vi "Dac_Output_cam_trig_multiple_digital_signals.vi"(0 "File to read":path=path "C:/Users/lpk27/Documents/pan-ASLMsynched/pan-ASLM/Calibration files/newcalibration_voice coil input_25msflyback.txt", 1 "Image acquisition time (ms)":dbl=1000.0, 2 "Delay between frames":dbl=25.0, 3 "Laser Toggles":T1 {"Laser 488 order selection" items=["Not active", "1", "2", "3", "4"]; "Laser 642 order selection" items=["Not active", "1", "2", "3", "4"]; "Laser 595 order selection" items=["Not active", "1", "2", "3", "4"]; "Laser 560 order selection" items=["Not active", "1", "2", "3", "4"]; "Laser 642 nm power" min=0.0 max=5.0 scale=0.0..100.0; "Laser 595 nm power" min=0.0 max=5.0 scale=0.0..100.0; "Laser 560 nm power" min=0.0 max=5.0 scale=0.0..100.0; "Laser 488 nm power" min=0.0 max=5.0 scale=0.0..100.0}, 4 "stop":bool, 5 "error in":errorcluster, 6 "Time Target (s)":dbl=-1.0, 11 "Setup":enum16{"Test setup", "Microscope"}(ring)) -> (19 "error out":errorcluster)   [LabVIEW 2020]
uses:
  typedefs/Laser_toggles_typedef.ctl
  <vilib>/DAQmx/write.llb/DAQmx Write (Digital Wfm 1Chan NSamp).vi
  <vilib>/DAQmx/write.llb/DAQmx Write (Analog Wfm 1Chan NSamp).vi
  <vilib>/Utility/file.llb/Read Delimited Spreadsheet (DBL).vi
  <vilib>/DAQmx/create/channels.llb/DAQmx Create Channel (AO-Voltage-Basic).vi
  <vilib>/DAQmx/configure/timing.llb/DAQmx Timing (Sample Clock).vi
  <vilib>/DAQmx/miscellaneous.llb/DAQmx Fill In Error Info.vi
  <vilib>/DAQmx/create/channels.llb/DAQmx Create Channel (CO-Pulse Generation-Ticks).vi
  <vilib>/DAQmx/configure/timing.llb/DAQmx Timing (Implicit).vi
  <vilib>/DAQmx/create/channels.llb/DAQmx Create Channel (DO-Digital Output).vi
  <vilib>/Waveform/DWDTOps.llb/DWDT Uncompress Digital.vi
  <vilib>/DAQmx/create/channels.llb/DAQmx Create Channel (CO-Pulse Generation-Frequency).vi
  Global stop DAQ.vi
  <resource>/objmgr/daqmx.rc
panel:
  out "error out 4":errorcluster
  out "error out 3":errorcluster
  out "error out 2":errorcluster
  out "Digital Waveform Graph":digitalwaveform(graph)
  out "LabVIEW generated Sawtooth input (blue) and Camera trigger (red)":waveform(dbl)(graph)={"t0"=timestamp(0 s since 1904-01-01), "dt"=1.0, "Y"=array[3075 elements]}
  out "# Samples written per channel":u32=3075
  out "actual frequency":dbl=1000.0
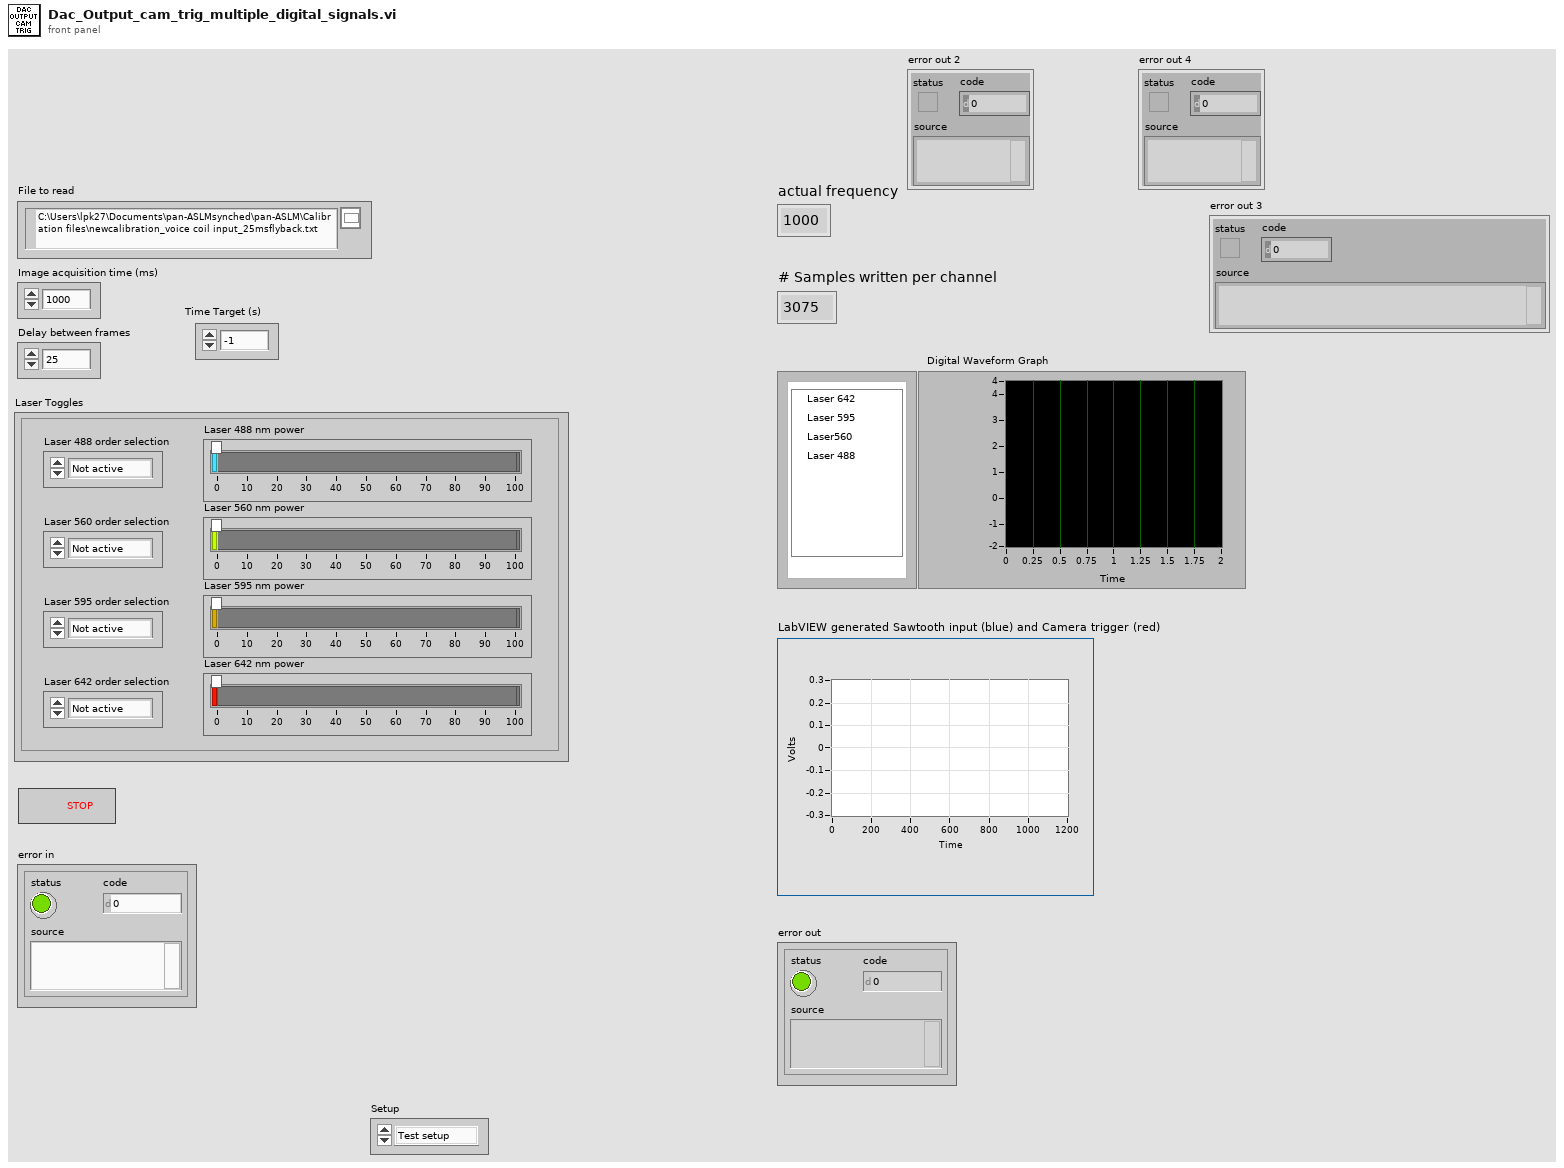
[diagram p1: front panel]
types:
  T1 = typedef "Laser_toggles_typedef.ctl" = cluster{"Laser 488 nm power":dbl, "Laser 560 nm power":dbl, "Laser 595 nm power":dbl, "Laser 642 nm power":dbl, "Laser 560 order selection":u16, "Laser 595 order selection":u16, "Laser 642 order selection":u16, "Laser 488 order selection":u16}
  T2 = typedef "DAQ_channel_typedef.ctl" = cluster{"CO.Pulse.Term":tag, "Voice coil analog output":tag, "counter":tag, "CO.Pulse.Term 2":tag, "AOTF lines":tag, "counter 2":tag, "CO.Pulse.Term 3":tag, "counter 3":tag}
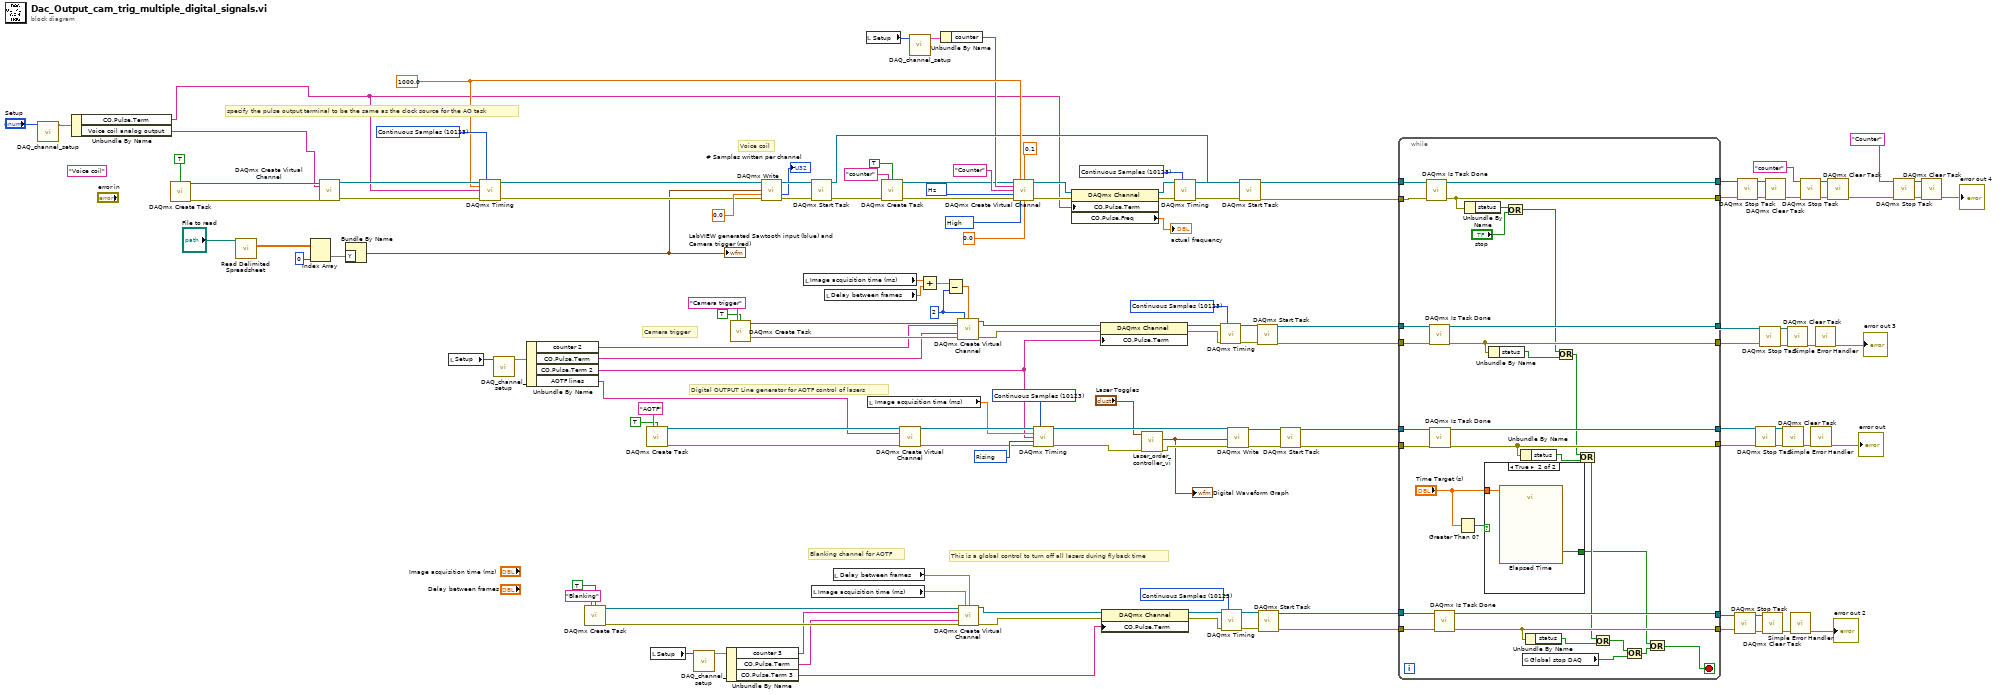
[diagram p0: block diagram]
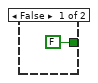
[diagram p2: hidden frame]
diagram:
  (unwired) "Voice coil" ("new task name")
  w86 = 10123 items=["Finite Samples"=10178, "Continuous Samples"=10123, "Hardware Timed Single Point"=12522] ("sample mode")
  w91 = 10123 items=["Finite Samples"=10178, "Continuous Samples"=10123, "Hardware Timed Single Point"=12522] ("sample mode")
  w99 = 10280 items=["Rising"=10280, "Falling"=10171] ("active edge")
  w71 = u32 2 ("high ticks")
  w109 = 10123 items=["Finite Samples"=10178, "Continuous Samples"=10123, "Hardware Timed Single Point"=12522] ("sample mode")
  w121 = 10192 items=["High"=10192, "Low"=10214] ("idle state")
  w122 = 10373 items=["Hz"=10373] ("units")
  w115 = 10123 items=["Finite Samples"=10178, "Continuous Samples"=10123, "Hardware Timed Single Point"=12522] ("sample mode")
  w114 = 1000.0 ("rate")
  w136 = 10123 items=["Finite Samples"=10178, "Continuous Samples"=10123, "Hardware Timed Single Point"=12522] ("sample mode")
  # "This is a global control to turn off all lasers during flyback time"
  # "Voice coil"
  # "Camera trigger"
  # "Digital OUTPUT Line generator for AOTF control of lasers"
  # "Blanking channel for AOTF"
  # "specify the pulse output terminal to be the same as the clock source for the AO task"
  n1 = call "DAQ_channel_setup.vi"("Text Ring"="Setup") -> ("DAQ channels OUT"=w24:T2)  [unwired: 10 in]
  n2 = Unbundle By Name(w24) -> ("CO.Pulse.Term"=w9:tag, "Voice coil analog output"=w25:tag)
  n3 = call <vilib>:"DAQmx Create Task.vi"("auto cleanup"=TRUE) -> ("task out"=w63:refnum<k21>, "error out"=w62:errorcluster)  [unwired: 13 in]
  n4 = call-poly <vilib>:"Read Delimited Spreadsheet.vi"("file path (dialog if empty)"="File to read") -> ("all rows"=w105:dbl[][])  [unwired: 9 in, 5 out]
  n5 = Index Array(array=w105, index (col)=0 ("disabled index (col)")) -> (element=w103:dbl[])  [unwired: 1 in]
  n6 = call-poly <vilib>:"DAQmx Create Virtual Channel.vi"("task in"=w63, "physical channels"=w25, "error in"=w62) -> ("task out"=w138:refnum<k21>, "error out"=w137:errorcluster)  [unwired: 11 in]
  n7 = Bundle By Name("Y"=w103) -> (w102:waveform(dbl))  [unwired: 1 in]
  "LabVIEW generated Sawtooth input (blue) and Camera trigger (red)" <- w102
  n8 = local read "Setup"() -> (w12:enum16{"Test setup", "Microscope"})
  n9 = call-poly <vilib>:"DAQmx Timing.vi"("task/channels in"=w138, "sample mode"=w136, "rate"=w114, "source"=w9, "error in"=w137) -> ("task out"=w117:refnum<k21>, "error out"=w116:errorcluster)  [unwired: 9 in]
  n10 = call "DAQ_channel_setup.vi"("Text Ring"=w12) -> ("DAQ channels OUT"=w21:T2)  [unwired: 10 in]
  n11 = Unbundle By Name(w21) -> ("counter 2"=w15:tag, "CO.Pulse.Term"=w5:tag, "CO.Pulse.Term 2"=w20:tag, "AOTF lines"=w19:tag)
  n12 = call <vilib>:"DAQmx Create Task.vi"("new task name"="Blanking", "auto cleanup"=TRUE) -> ("task out"=w68:refnum<k21>, "error out"=w67:errorcluster)  [unwired: 12 in]
  n13 = call <vilib>:"DAQmx Create Task.vi"("new task name"="AOTF", "auto cleanup"=TRUE) -> ("task out"=w65:refnum<k21>, "error out"=w64:errorcluster)  [unwired: 12 in]
  n14 = local read "Setup"() -> (w13:enum16{"Test setup", "Microscope"})
  n15 = call "DAQ_channel_setup.vi"("Text Ring"=w13) -> ("DAQ channels OUT"=w18:T2)  [unwired: 10 in]
  n16 = Unbundle By Name(w18) -> ("counter 3"=w17:tag, "CO.Pulse.Term"=w4:tag, "CO.Pulse.Term 3"=w16:tag)
  n17 = call <vilib>:"DAQmx Create Task.vi"("new task name"="Camera trigger", "auto cleanup"=TRUE) -> ("task out"=w59:refnum<k21>, "error out"=w60:errorcluster)  [unwired: 12 in]
  n18 = call-poly <vilib>:"DAQmx Write.vi"("task/channels in"=w117, "data"=w102, "timeout"=0.0, "error in"=w116) -> ("task out"=w126:refnum<k21>, "number of samples written per channel"=→"# Samples written per channel":u32, "error out"=w125:errorcluster)  [unwired: 9 in]
  n19 = local read "Image acquisition time (ms)"() -> (w74:dbl)
  n20 = call <vilib>:"DAQmx Start Task.vi"("task/channels in"=w126, "error in"=w125) -> ("task out"=w30:refnum<k21>, "error out"=w120:errorcluster)  [unwired: 12 in]
  n21 = local read "Image acquisition time (ms)"() -> (w76:dbl)
  n22 = local read "Delay between frames"() -> (w73:dbl)
  n23 = local read "Delay between frames"() -> (w75:dbl)
  n24 = local read "Setup"() -> (w11:enum16{"Test setup", "Microscope"})
  n25 = local read "Image acquisition time (ms)"() -> (w81:dbl)
  n26 = call <vilib>:"DAQmx Create Task.vi"("new task name"="counter", "auto cleanup"=TRUE, "error in"=w120) -> ("task out"=w7:refnum<k21>, "error out"=w133:errorcluster)  [unwired: 11 in]
  n27 = call-poly <vilib>:"DAQmx Create Virtual Channel.vi"("task in"=w65, "lines"=w19, "error in"=w64) -> ("task out"=w98:refnum<k21>, "error out"=w97:errorcluster)  [unwired: 11 in]
  n28 = call "DAQ_channel_setup.vi"("Text Ring"=w11) -> ("DAQ channels OUT"=w23:T2)  [unwired: 10 in]
  n29 = Add(x=w74, y=w73) -> (x+y=w72:dbl)
  n30 = Unbundle By Name(w23) -> ("counter"=w22:tag)
  n31 = Subtract(x=w72, y=w71) -> (x-y=w70:dbl)
  n32 = call-poly <vilib>:"DAQmx Create Virtual Channel.vi"("task in"=w59, "high ticks"=w71, "low ticks"=w70, "counter"=w15, "source of ticks"=w5, "error in"=w60) -> ("task out"=w113:refnum<k21>, "error out"=w101:errorcluster)  [unwired: 8 in]
  n33 = call-poly <vilib>:"DAQmx Create Virtual Channel.vi"("task in"=w68, "high ticks"=w76, "low ticks"=w75, "counter"=w17, "source of ticks"=w4, "error in"=w67) -> ("task out"=w90:refnum<k21>, "error out"=w83:errorcluster)  [unwired: 8 in]
  n34 = call-poly <vilib>:"DAQmx Create Virtual Channel.vi"("task in"=w7, "frequency"=w114, "duty cycle"=0.1, "counter"=w22, "name to assign"="Counter", "units"=w122, "error in"=w133, "idle state"=w121, "initial delay"=0.0) -> ("task out"=w132:refnum<k21>, "error out"=w131:errorcluster)  [unwired: 5 in]
  n35 = call-poly <vilib>:"DAQmx Timing.vi"("task/channels in"=w98, "sample mode"=w91, "rate"=w81, "source"=w20, "active edge"=w99, "error in"=w97) -> ("task out"=w94:refnum<k21>, "error out"=w79:errorcluster)  [unwired: 8 in]
  n36 = property class="DAQmx Channel"(reference=w132, error in=w131, "CO.Pulse.Term"=w9) -> (reference out=w128:refnum<k21>, error out=w129:errorcluster, "CO.Pulse.Freq"=→"actual frequency":dbl)
  n37 = property class="DAQmx Channel"(reference=w113, error in=w101, "CO.Pulse.Term"=w20) -> (reference out=w100:refnum<k21>, error out=w110:errorcluster)
  n38 = property class="DAQmx Channel"(reference=w90, error in=w83, "CO.Pulse.Term"=w16) -> (reference out=w82:refnum<k21>, error out=w87:errorcluster)
  n39 = call "Laser_order_controller_vi.vi"("error in"=w79, "Laser Toggles"="Laser Toggles") -> ("error out"=w78:errorcluster, "Digital Waveform Graph"=w77:digitalwaveform)  [unwired: 7 in, 1 out]
  "Digital Waveform Graph" <- w77
  n40 = call-poly <vilib>:"DAQmx Timing.vi"("task/channels in"=w128, "sample mode"=w115, "error in"=w129) -> ("task out"=w135:refnum<k21>, "error out"=w134:errorcluster)  [unwired: 11 in]
  n41 = call-poly <vilib>:"DAQmx Timing.vi"("task/channels in"=w100, "sample mode"=w109, "error in"=w110) -> ("task out"=w108:refnum<k21>, "error out"=w107:errorcluster)  [unwired: 11 in]
  n42 = call-poly <vilib>:"DAQmx Timing.vi"("task/channels in"=w82, "sample mode"=w86, "error in"=w87) -> ("task out"=w85:refnum<k21>, "error out"=w84:errorcluster)  [unwired: 11 in]
  n43 = call-poly <vilib>:"DAQmx Write.vi"("task/channels in"=w94, "data"=w77, "error in"=w78) -> ("task out"=w96:refnum<k21>, "error out"=w95:errorcluster)  [unwired: 10 in, 1 out]
  n44 = call <vilib>:"DAQmx Start Task.vi"("task/channels in"=w135, "error in"=w134) -> ("error out"=w127:errorcluster)  [unwired: 12 in, 1 out]
  n45 = call <vilib>:"DAQmx Start Task.vi"("task/channels in"=w108, "error in"=w107) -> ("task out"=w112:refnum<k21>, "error out"=w111:errorcluster)  [unwired: 12 in]
  n46 = call <vilib>:"DAQmx Start Task.vi"("task/channels in"=w85, "error in"=w84) -> ("task out"=w89:refnum<k21>, "error out"=w88:errorcluster)  [unwired: 12 in]
  n47 = call <vilib>:"DAQmx Start Task.vi"("task/channels in"=w96, "error in"=w95) -> ("task out"=w93:refnum<k21>, "error out"=w92:errorcluster)  [unwired: 12 in]
  n48 = while {
    tunnel: w127 -> [w169]
    tunnel: w30 -> [w168]
    tunnel: w112 -> [w167]
    tunnel: w111 -> [w166]
    tunnel: w93 -> [w165]
    tunnel: w92 -> [w164]
    tunnel: w89 -> [w163]
    tunnel: w88 -> [w162]
    tunnel: [w161] -> w44
    tunnel: [w152] -> w43
    tunnel: [w160] -> w49
    tunnel: [w159] -> w48
    tunnel: [w158] -> w38
    tunnel: [w157] -> w37
    tunnel: [w156] -> w36
    tunnel: [w155] -> w35
    stop <- w142 stop-if-true
    n49 = call <vilib>:"DAQmx Is Task Done.vi"("task/channels in"=w168, "error in"=w169) -> ("task out"=w161:refnum<k21>, "error out"=w152:errorcluster)  [unwired: 11 in, 1 out]
    n50 = call <vilib>:"DAQmx Is Task Done.vi"("task/channels in"=w167, "error in"=w166) -> ("task out"=w160:refnum<k21>, "error out"=w159:errorcluster)  [unwired: 11 in, 1 out]
    n51 = call <vilib>:"DAQmx Is Task Done.vi"("task/channels in"=w165, "error in"=w164) -> ("task out"=w158:refnum<k21>, "error out"=w157:errorcluster)  [unwired: 11 in, 1 out]
    n52 = call <vilib>:"DAQmx Is Task Done.vi"("task/channels in"=w163, "error in"=w162) -> ("task out"=w156:refnum<k21>, "error out"=w155:errorcluster)  [unwired: 11 in, 1 out]
    n53 = Greater Than 0?(x="Time Target (s)") -> (x > 0?=w140:bool)
    n54 = Unbundle By Name(w152) -> ("status"=w146:bool)
    n55 = case shown="True" w140 {
      tunnel: [FALSE ("Time has Elapsed") w172] -> w141
      tunnel: "Time Target (s)" -> [_ w171]
      frame False {
      }
      frame True {
        n56 = call "Elapsed Time"("Time Target (s)"=w171) -> ("Time has Elapsed"=w172:bool)  [unwired: 11 in, 7 out]
      }
    }
    n57 = Unbundle By Name(w159) -> ("status"=w151:bool)
    n58 = Or(x=w146, y="stop") -> (x .or. y?=w144:bool)
    n59 = Unbundle By Name(w157) -> ("status"=w150:bool)
    n60 = global read "Global stop DAQ.vi" "Global stop DAQ"() -> (w147:bool)
    n61 = Unbundle By Name(w155) -> ("status"=w148:bool)
    n62 = Or(x=w144, y=w151) -> (x .or. y?=w154:bool)
    n63 = Or(x=w154, y=w150) -> (x .or. y?=w153:bool)
    n64 = Or(x=w153, y=w148) -> (x .or. y?=w149:bool)
    n65 = Or(x=w149, y=w147) -> (x .or. y?=w143:bool)
    n66 = Or(x=w141, y=w143) -> (x .or. y?=w142:bool)
  }
  n67 = call <vilib>:"DAQmx Stop Task.vi"("task/channels in"=w36, "error in"=w35) -> ("task out"=w33:refnum<k21>, "error out"=w34:errorcluster)  [unwired: 12 in]
  n68 = call <vilib>:"DAQmx Stop Task.vi"("task/channels in"=w44, "error in"=w43) -> ("task out"=w47:refnum<k21>, "error out"=w46:errorcluster)  [unwired: 12 in]
  n69 = call <vilib>:"DAQmx Stop Task.vi"("task/channels in"=w38, "error in"=w37) -> ("task out"=w41:refnum<k21>, "error out"=w42:errorcluster)  [unwired: 12 in]
  n70 = call <vilib>:"DAQmx Stop Task.vi"("task/channels in"=w49, "error in"=w48) -> ("task out"=w52:refnum<k21>, "error out"=w53:errorcluster)  [unwired: 12 in]
  n71 = call <vilib>:"DAQmx Clear Task.vi"("task in"=w33, "error in"=w34) -> ("error out"=w32:errorcluster)  [unwired: 13 in]
  n72 = call <vilib>:"DAQmx Clear Task.vi"("task in"=w47, "error in"=w46) -> ("error out"=w27:errorcluster)  [unwired: 13 in]
  n73 = call <vilib>:"DAQmx Clear Task.vi"("task in"=w41, "error in"=w42) -> ("error out"=w40:errorcluster)  [unwired: 13 in]
  n74 = call <vilib>:"DAQmx Clear Task.vi"("task in"=w52, "error in"=w53) -> ("error out"=w51:errorcluster)  [unwired: 13 in]
  n75 = call <vilib>:"Simple Error Handler.vi"("error in (no error)"=w32) -> ("error out"=→"error out 2":errorcluster)  [unwired: 4 in, 4 out]
  n76 = call <vilib>:"DAQmx Stop Task.vi"("task/channels in"="counter" ("new task name"), "error in"=w27) -> ("task out"=w29:refnum<k21>, "error out"=w28:errorcluster)  [unwired: 12 in]
  n77 = call <vilib>:"Simple Error Handler.vi"("error in (no error)"=w40) -> ("error out"=→"error out":errorcluster)  [unwired: 4 in, 4 out]
  n78 = call <vilib>:"Simple Error Handler.vi"("error in (no error)"=w51) -> ("error out"=→"error out 3":errorcluster)  [unwired: 4 in, 4 out]
  n79 = call <vilib>:"DAQmx Clear Task.vi"("task in"=w29, "error in"=w28) -> ("error out"=w26:errorcluster)  [unwired: 13 in]
  n80 = call <vilib>:"DAQmx Stop Task.vi"("task/channels in"="Counter" ("new task name"), "error in"=w26) -> ("task out"=w2:refnum<k21>, "error out"=w3:errorcluster)  [unwired: 12 in]
  n81 = call <vilib>:"DAQmx Clear Task.vi"("task in"=w2, "error in"=w3) -> ("error out"=→"error out 4":errorcluster)  [unwired: 13 in]
